vi "NewGame.vi"(8 "error in (no error)":errorcluster, 10 "Engine in":refnum<class "Engine.lvclass">, 11 "AttractScreenType (ChildObject)":refnum<class "AttractScreen.lvclass">) -> (0 "error out":errorcluster, 2 "Engine out":refnum<class "Engine.lvclass">, 3 "AttractScreen out":refnum<class "AttractScreen.lvclass">)   [LabVIEW 2019, in "RT_Game.lvlib" / "AttractScreen.lvclass"]
uses:
  AttractScreen.lvclass
  C:/Users/FreshBob/Dropbox/VIs/myRIO_GameConsole/RT/RT_Game/Game/Game.lvclass
  Engine/Engine.lvclass
  Direction.ctl
  SnakeDemo/SnakeDemo.lvclass
  PongDemo/PongDemo.lvclass
  BounceDemo/BounceDemo.lvclass
  Game/Game.lvclass/Game.ctl
  AttractScreen.lvclass/AttractScreen.ctl
  Game/Write ResetCameraOnLoad_.vi
  Game/Write HasHighscore_.vi
  Game/Write HasMenu_.vi
  Game/Game.lvclass
  RT_Game.lvlib
  Initializers/Initializers.lvlib
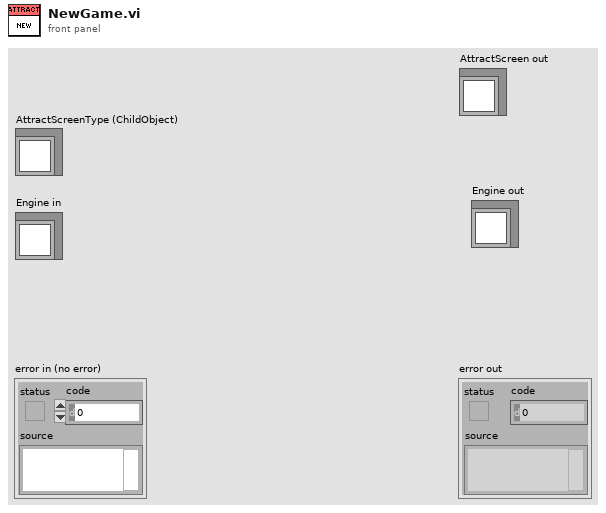
[diagram p1: front panel]
types:
  T1 = typedef "RT_Game.lvlib/Direction.ctl" = enum16{"none", "Both", "left", "right", "up", "down"}
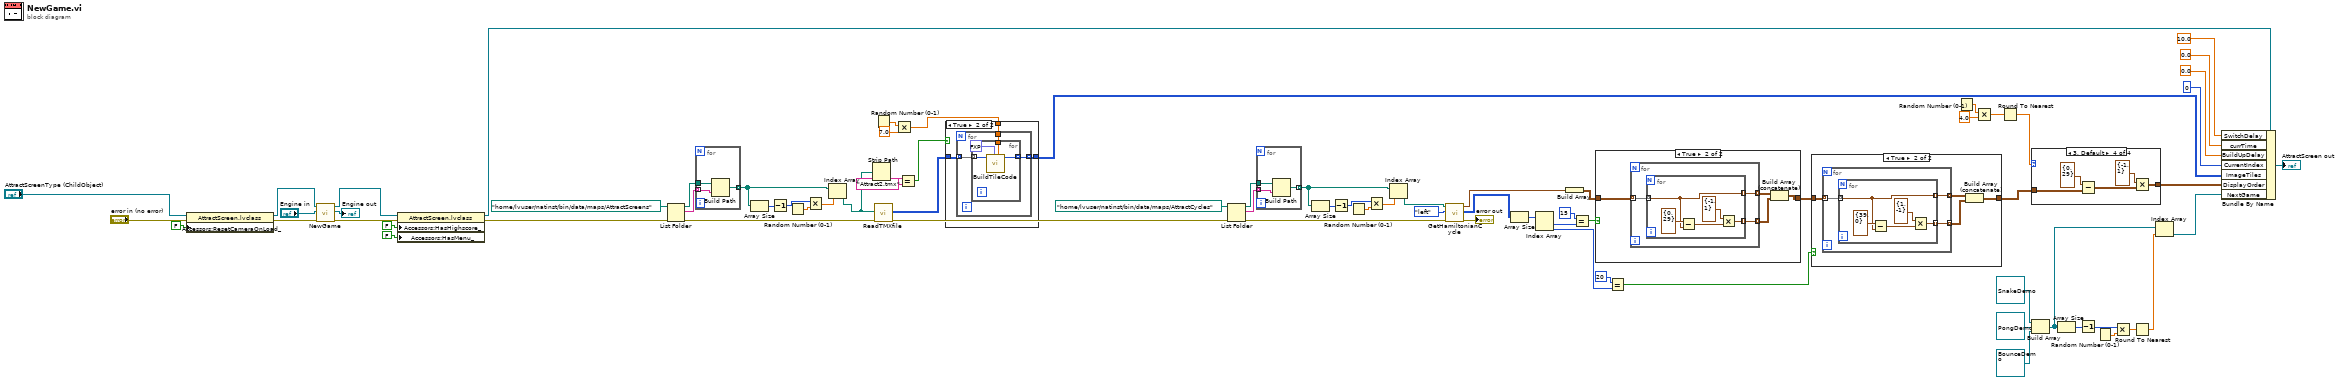
[diagram p0: block diagram]
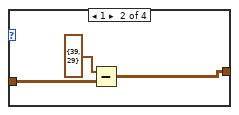
[diagram p6: hidden frame]
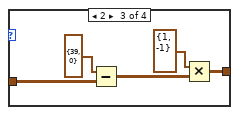
[diagram p7: hidden frame]
diagram:
  n1 = property class="AttractScreen.lvclass"(reference="AttractScreenType (ChildObject)", error in="error in (no error)", "Accessors:ResetCameraOnLoad_"=FALSE ("ResetCameraOnLoad_")) -> (reference out=w37:refnum<class "AttractScreen.lvclass">, error out=w39:errorcluster)
  n2 = call-parent "NewGame.vi"("error in (no error)"=w39, "Engine in"="Engine in", "GameType (ChildObject)"=w37) -> ("error out"=w76:errorcluster, "Engine out"=→"Engine out":refnum<class "Engine.lvclass">, "Game out"=w69:refnum<class "AttractScreen.lvclass">)  [unwired: 6 in]
  n3 = property class="AttractScreen.lvclass"(reference=w69, error in=w76, "Accessors:HasHighscore_"=FALSE ("HasHighscore_"), "Accessors:HasMenu_"=FALSE ("HasMenu_")) -> (reference out=w68:refnum<class "AttractScreen.lvclass">, error out=w70:errorcluster)
  n4 = List Folder(path=path "/home/lvuser/natinst/bin/data/maps/AttractScreens" ("path to tmx-file (created with Tiles2D)"), error in=w70) -> (path out=w59:path, filenames=w58:string[], error out=w61:errorcluster)  [unwired: 2 in, 1 out]
  n5 = for {
    tunnel: w59 -> [w79]
    tunnel: w58 -> [w78] mode=indexing
    tunnel: [w77] -> w54 mode=indexing
    n6 = Build Path(base path=w79, name or relative path=w78) -> (appended path=w77:path)
  }
  n7 = Array Size(array=w54) -> (size(s)=w57:i32)
  n8 = Decrement(x=w57) -> (x-1=w56:i32)
  n9 = Random Number (0-1)() -> (number: 0 to 1=w55:dbl)
  n10 = Multiply(x=w56, y=w55) -> (x*y=w53:dbl)
  n11 = Index Array(array=w54, index=w53) -> (element=w9:path)
  n12 = Strip Path(path=w9) -> (name=w8:string)  [unwired: 1 out]
  n13 = call "ReadTMXfile.vi"("error in (no error)"=w61, "path to tmx-file (created with Tiles2D)"=w9) -> ("error out"=w44:errorcluster, "Tilenumbers"=w6:u32[][])  [unwired: 8 in]
  n14 = Random Number (0-1)() -> (number: 0 to 1=w3:dbl)
  n15 = Multiply(x=w3, y=7.0) -> (x*y=w1:dbl)
  n16 = Equal?(x=w8, y="Attract2.tmx") -> (x = y?=w4:bool)
  n17 = case shown="True" w4 {
    tunnel: w6 -> [w80 w83]
    tunnel: [w80 w82] -> w5
    tunnel: w1 -> [_ w81]
    frame False {
    }
    frame True {
      n18 = for {
        tunnel: w83 -> [w86] mode=indexing
        tunnel: [w85] -> w82 mode=indexing
        tunnel: w81 -> [w84]
        n19 = for {
          tunnel: w86 -> [w90] mode=indexing
          tunnel: [w89] -> w85 mode=indexing
          tunnel: w84 -> [w87]
          n20 = call "BuildTileCode.vi"("replacecolor"=w87, "color_to_replace"=fxp<+,3,3> 2.0, "Tilenumber"=w90) -> ("Tilecode"=w89:u32)  [unwired: 8 in]
        }
      }
    }
  }
  n21 = List Folder(path=path "/home/lvuser/natinst/bin/data/maps/AttractCycles" ("path to tmx-file (created with Tiles2D)"), error in=w44) -> (path out=w46:path, filenames=w47:string[], error out=w42:errorcluster)  [unwired: 2 in, 1 out]
  n22 = for {
    tunnel: w46 -> [w93]
    tunnel: w47 -> [w92] mode=indexing
    tunnel: [w91] -> w51 mode=indexing
    n23 = Build Path(base path=w93, name or relative path=w92) -> (appended path=w91:path)
  }
  n24 = Array Size(array=w51) -> (size(s)=w48:i32)
  n25 = Decrement(x=w48) -> (x-1=w49:i32)
  n26 = Random Number (0-1)() -> (number: 0 to 1=w50:dbl)
  n27 = Multiply(x=w49, y=w50) -> (x*y=w52:dbl)
  n28 = Index Array(array=w51, index=w52) -> (element=w41:path)
  n29 = call "GetHamiltonianCycle.vi"("error in (no error)"=w42, "StartDir (up)"=Direction."left", "path to tmx-file (created with Tiles2D)"=w41) -> ("error out"=→"error out":errorcluster, "Hamilton2D"=w21:u32[][], "Hamilton1D"=w71:cluster{i32, i32}[])  [unwired: 5 in, 1 out]
  n30 = Array Size(array=w21) -> (size(s)=w20:i32[])
  n31 = Index Array(array=w20) -> (element #1=w19:i32, element #2=w12:i32)  [unwired: 2 in]
  n32 = Build Array(w71) -> (w16:cluster{i32, i32}[][])
  n33 = Equal?(x=15, y=w19) -> (x = y?=w17:bool)
  n34 = case shown="True" w17 {
    tunnel: w16 -> [w94 w98]
    tunnel: [w94 w96] -> w15
    frame False {
    }
    frame True {
      n35 = for {
        tunnel: w98 -> [w101] mode=indexing
        tunnel: [w100] -> w97 mode=indexing
        tunnel: [w99] -> w95 mode=indexing
        n36 = for {
          tunnel: w101 -> [w103] mode=indexing
          tunnel: [w103] -> w100 mode=indexing
          tunnel: [w102] -> w99 mode=indexing
          n37 = Subtract(x=cluster{i32, i32} {0, 29}, y=w103) -> (x-y=w104:cluster{i32, i32})
          n38 = Multiply(x=cluster{i32, i32} {-1, 1}, y=w104) -> (x*y=w102:cluster{i32, i32})
        }
      }
      n39 = Build Array (concatenate)(w97, w95) -> (w96:cluster{i32, i32}[][])
    }
  }
  n40 = Equal?(x=20, y=w12) -> (x = y?=w11:bool)
  n41 = case shown="True" w11 {
    tunnel: w15 -> [w107 w111]
    tunnel: [w107 w109] -> w14
    frame False {
    }
    frame True {
      n42 = for {
        tunnel: w111 -> [w114] mode=indexing
        tunnel: [w113] -> w110 mode=indexing
        tunnel: [w112] -> w108 mode=indexing
        n43 = for {
          tunnel: w114 -> [w116] mode=indexing
          tunnel: [w116] -> w113 mode=indexing
          tunnel: [w115] -> w112 mode=indexing
          n44 = Subtract(x=cluster{i32, i32} {39, 0}, y=w116) -> (x-y=w117:cluster{i32, i32})
          n45 = Multiply(x=cluster{i32, i32} {1, -1}, y=w117) -> (x*y=w115:cluster{i32, i32})
        }
      }
      n46 = Build Array (concatenate)(w110, w108) -> (w109:cluster{i32, i32}[][])
    }
  }
  n47 = Random Number (0-1)() -> (number: 0 to 1=w25:dbl)
  n48 = Multiply(x=w25, y=4.0) -> (x*y=w23:dbl)
  n49 = Round To Nearest(number=w23) -> (nearest integer value=w22:dbl)
  n50 = case shown="3, Default" w22 {
    tunnel: w14 -> [w120 w123 w128 w133]
    tunnel: [w120 w122 w125 w130] -> w26
    frame 0 {
    }
    frame 1 {
      n51 = Subtract(x=cluster{i32, i32} {39, 29}, y=w123) -> (x-y=w122:cluster{i32, i32}[][])
    }
    frame 2 {
      n52 = Subtract(x=cluster{i32, i32} {39, 0}, y=w128) -> (x-y=w127:cluster{i32, i32}[][])
      n53 = Multiply(x=cluster{i32, i32} {1, -1}, y=w127) -> (x*y=w125:cluster{i32, i32}[][])
    }
    frame 3, Default {
      n54 = Subtract(x=cluster{i32, i32} {0, 29}, y=w133) -> (x-y=w132:cluster{i32, i32}[][])
      n55 = Multiply(x=cluster{i32, i32} {-1, 1}, y=w132) -> (x*y=w130:cluster{i32, i32}[][])
    }
  }
  n56 = Build Array(refnum<class "SnakeDemo.lvclass"> refnum ("RT_Game.lvlib:SnakeDemo.lvclass"), refnum<class "PongDemo.lvclass"> refnum ("RT_Game.lvlib:PongDemo.lvclass"), refnum<class "BounceDemo.lvclass"> refnum ("RT_Game.lvlib:BounceDemo.lvclass")) -> (w34:refnum<class "Game.lvclass">[])
  n57 = Array Size(array=w34) -> (size(s)=w30:i32)
  n58 = Decrement(x=w30) -> (x-1=w35:i32)
  n59 = Random Number (0-1)() -> (number: 0 to 1=w31:dbl)
  n60 = Multiply(x=w35, y=w31) -> (x*y=w32:dbl)
  n61 = Round To Nearest(number=w32) -> (nearest integer value=w33:dbl)
  n62 = Index Array(array=w34, index=w33) -> (element=w27:refnum<class "Game.lvclass">)
  n63 = Bundle By Name(cluster=w68, "SwitchDelay"=10.0, "currTime"=0.0, "BuildUpDelay"=0.0 ("Delay"), "CurrentIndex"=i16 0, "ImageTiles"=w5, "DisplayOrder"=w26, "NextGame"=w27) -> (→"AttractScreen out":refnum<class "AttractScreen.lvclass">)
